vi "sensor.vi"() -> (0 "Numeric":dbl)   [LabVIEW 2022 SP3]
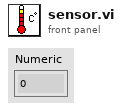
[diagram p1: front panel]
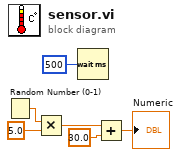
[diagram p0: block diagram]
diagram:
  n1 = Random Number (0-1)() -> (number: 0 to 1=w5:dbl)
  n2 = Multiply(x=w5, y=5.0) -> (x*y=w3:dbl)
  n3 = Wait (ms)(milliseconds to wait=u32 500) -> ()  [unwired: 1 out]
  n4 = Add(x=w3, y=30.0 ("x+y")) -> (x+y=→"Numeric":dbl)
